vi "Shooter Button SUBVI.vi"   [LabVIEW 2013]
types:
  T1 = cluster{"Digital Input [1-16][0]":bool, "Digital Input [1-16][1]":bool, "Digital Input [1-16][2]":bool, "Digital Input [1-16][3]":bool, "Digital Input [1-16][4]":bool, "Digital Input [1-16][5]":bool, "Digital Input [1-16][6]":bool, "Digital Input [1-16][7]":bool, "Digital Input [1-16][8]":bool, "Digital Input [1-16][9]":bool, "Digital Input [1-16][10]":bool, "Digital Input [1-16][11]":bool, "Digital Input [1-16][12]":bool, "Digital Input [1-16][13]":bool, "Digital Input [1-16][14]":bool, "Digital Input [1-16][15]":bool}
  T2 = typedef "WPI_DigitalInputDevRef.ctl" = cluster{"DevStatus":errorcluster, "DIO Channel":T3, "Digital Module":T4}
  T3 = typedef "FPGA_DIOChannel.ctl" = enum8{"DIO 1", "DIO 2", "DIO 3", "DIO 4", "DIO 5", "DIO 6", "DIO 7", "DIO 8", "DIO 9", "DIO 10", "DIO 11", "DIO 12", "DIO 13", "DIO 14", "Invalid"}
  T4 = typedef "FPGA_TypedefDigitalModule.ctl" = enum16{"Digital Module 1", "Digital Module 2"}
  T5 = typedef "WPI_MotorControlDeviceRef.ctl" = cluster{"DeviceStatus":errorcluster, "Type":enum16{"PWM", "CAN"}, "PWM":cluster{"Digital Module":T4, "PWM Channel":T6, "DeadBand":T7}, "CAN":cluster{"Device Number":u8, "Control Mode":T8, "Semaphore":T9, "Max Vout":dbl}, "Invert":bool, "TransformRef":T10, "InvTransformRef":T10}
  T6 = typedef "FPGA_DIOPWMChannel.ctl" = enum8{"PWM 1", "PWM 2", "PWM 3", "PWM 4", "PWM 5", "PWM 6", "PWM 7", "PWM 8", "PWM 9", "PWM 10", "Invalid"}
  T7 = typedef "WPI_PWMDeadband.ctl" = cluster{"Name":string, "maxPositivePwm":i32, "minPositivePwm":i32, "centerPwm":i32, "maxNegativePwm":i32, "minNegativePwm":i32, "angularRange":u16}
  T8 = typedef "WPI_CANJaguar_ControlMode.ctl" = enum8{"Percent VBus", "Current", "Speed", "Position", "Voltage"}
  T9 = typedef "Semaphore RefNum" = refnum<k1>
  T10 = typedef "WPI_PWMTransform_ConPane.ctl" = refnum<vi>
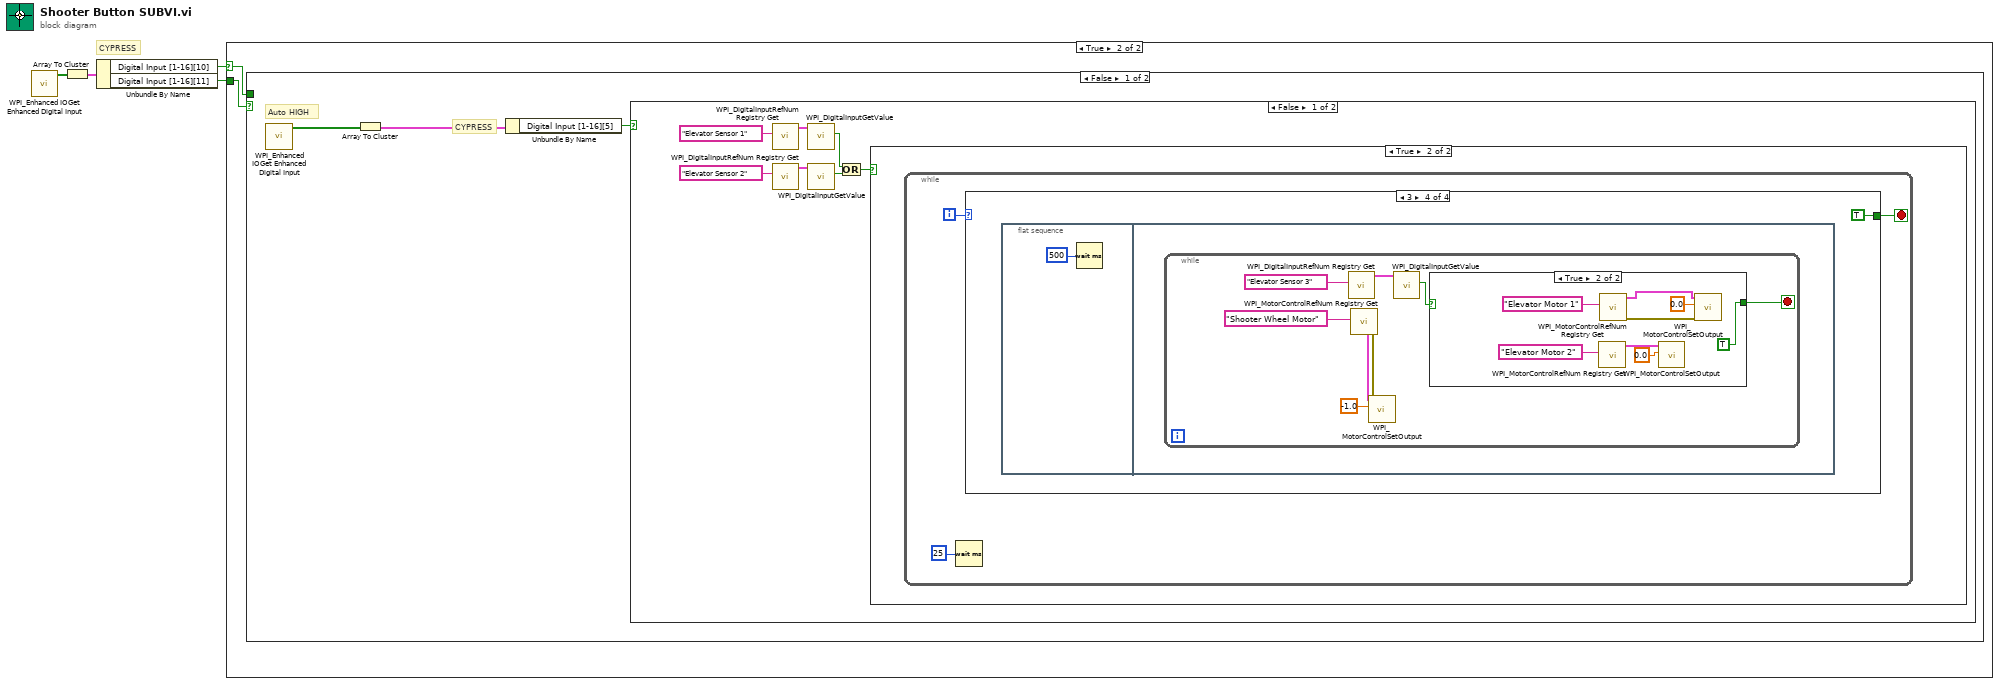
[diagram p0: block diagram]
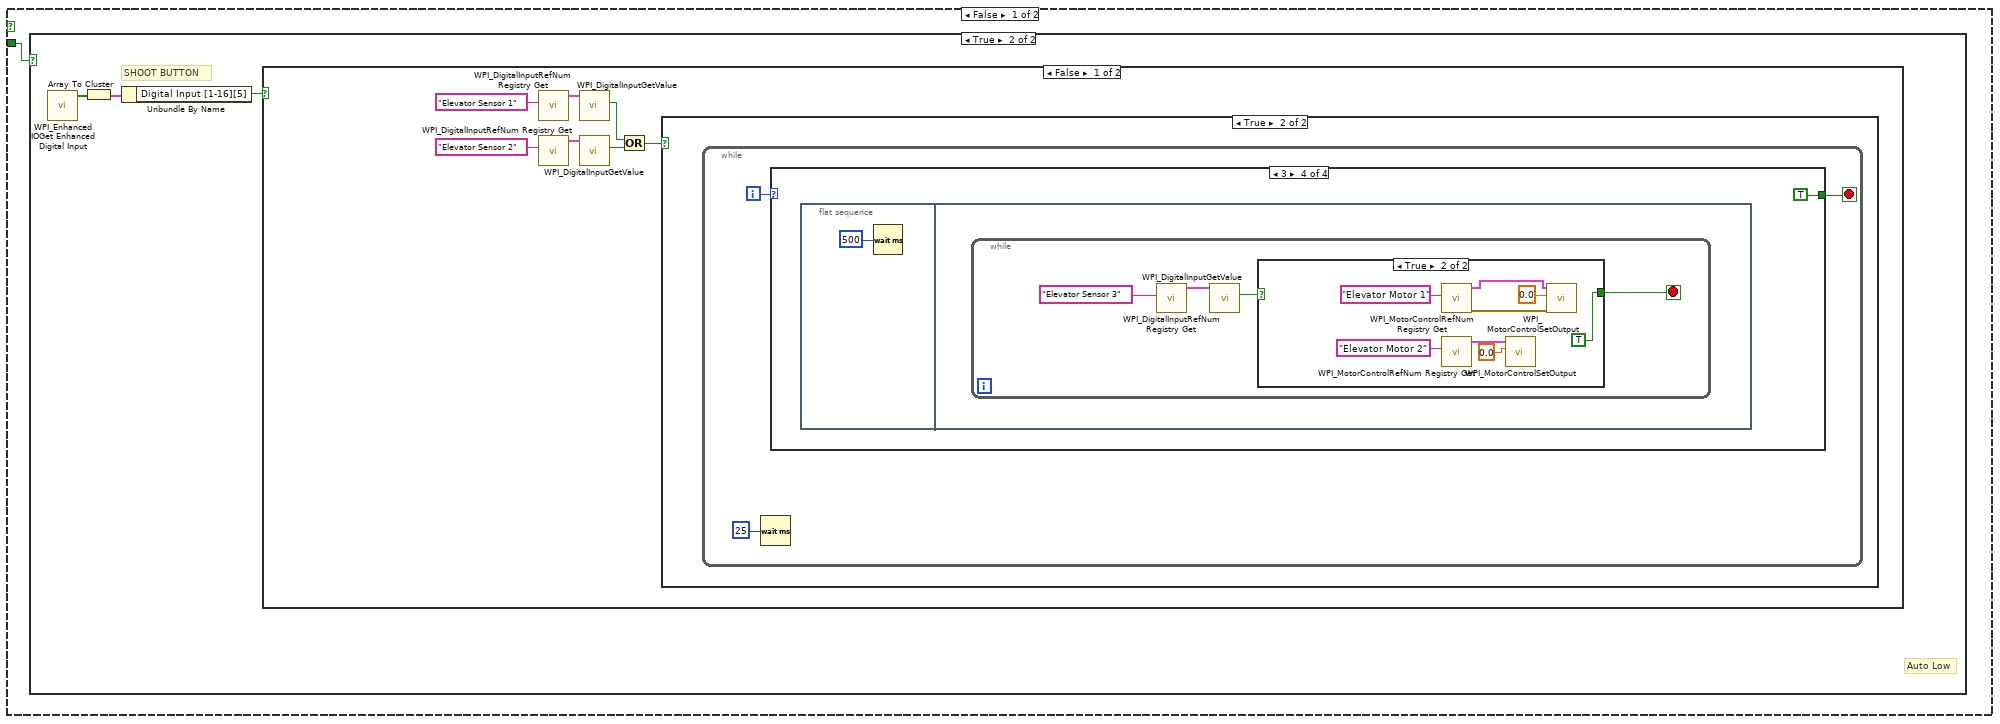
[diagram p2: hidden frame]
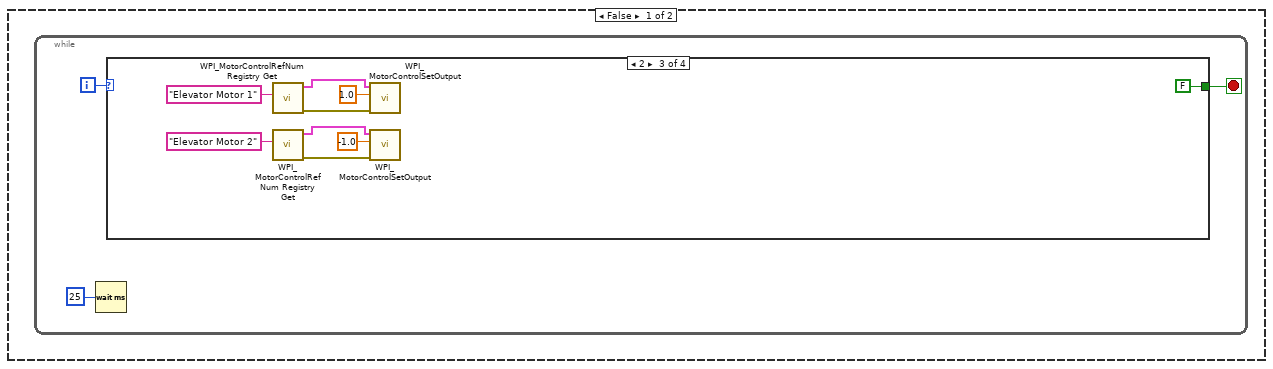
[diagram p4: hidden frame]
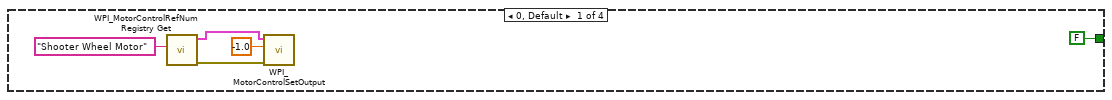
[diagram p5: hidden frame]
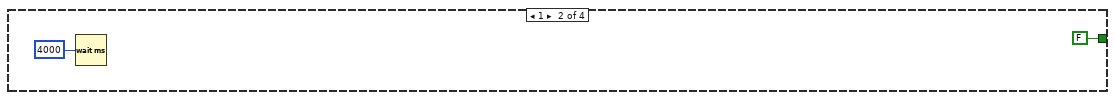
[diagram p6: hidden frame]
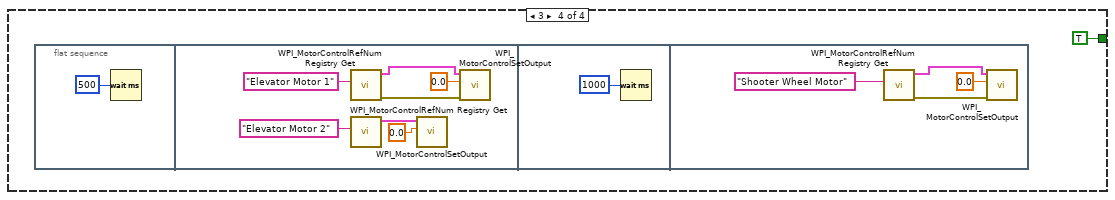
[diagram p7: hidden frame]
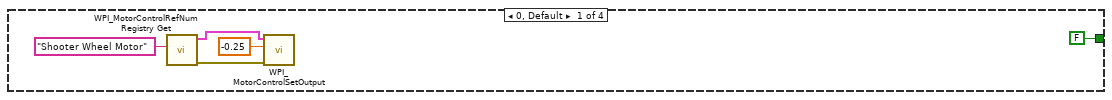
[diagram p8: hidden frame]
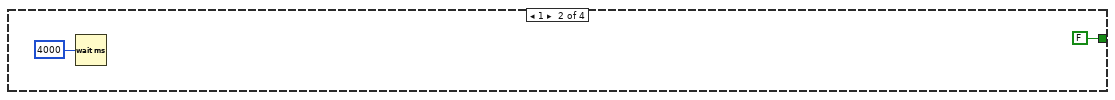
[diagram p9: hidden frame]
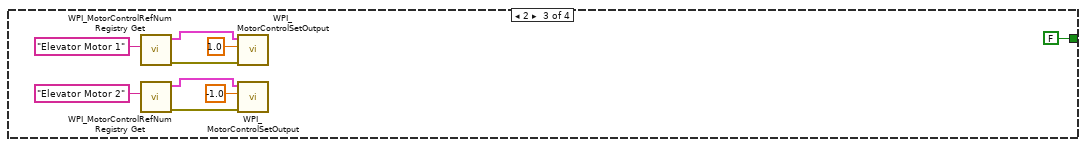
[diagram p10: hidden frame]
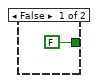
[diagram p11: hidden frame]
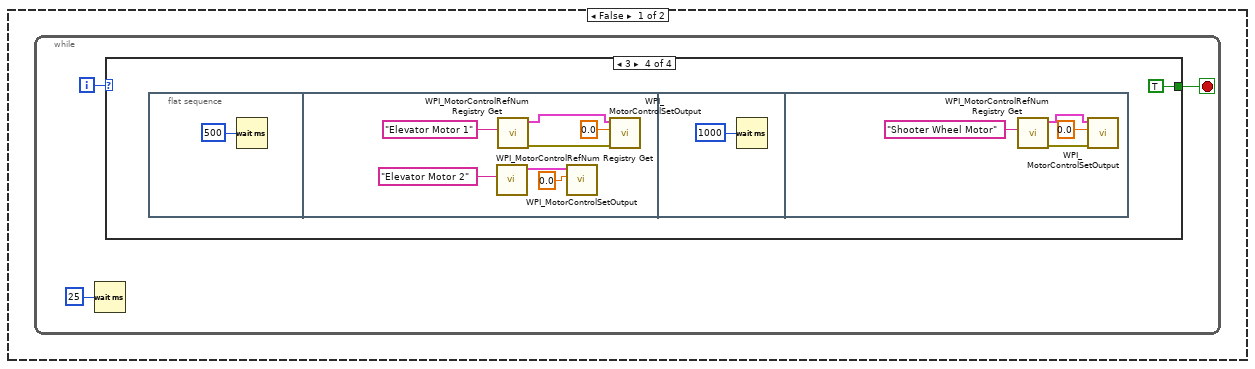
[diagram p13: hidden frame]
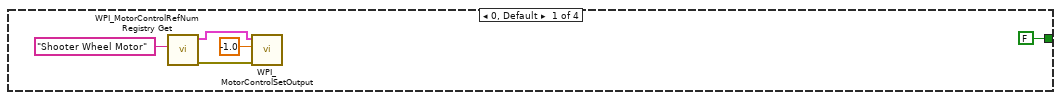
[diagram p14: hidden frame]
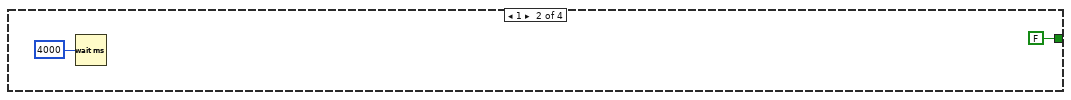
[diagram p15: hidden frame]
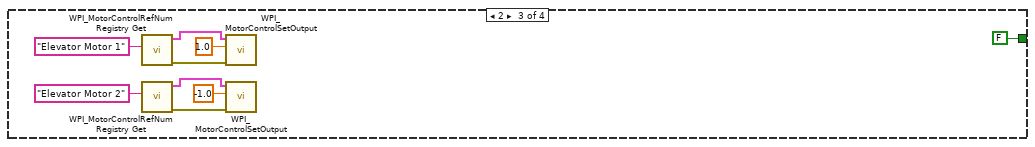
[diagram p16: hidden frame]
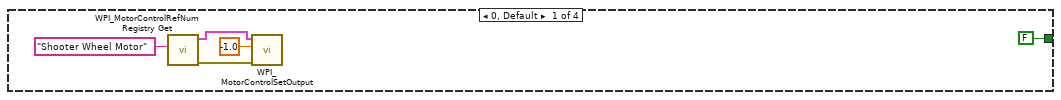
[diagram p17: hidden frame]
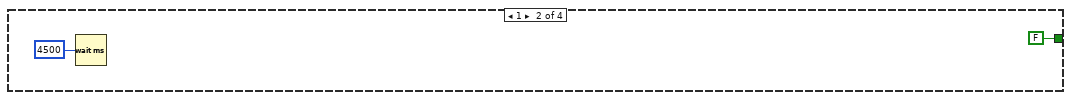
[diagram p18: hidden frame]
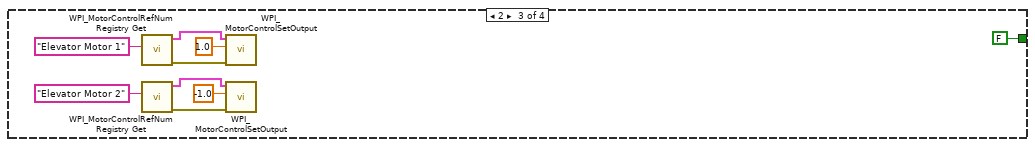
[diagram p19: hidden frame]
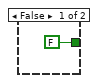
[diagram p20: hidden frame]
diagram:
  # "CYPRESS"
  n1 = call <vilib>:"WPI_Enhanced IOGet Enhanced Digital Input.vi"() -> ("Digital Input [1-16]"=w4:bool[])  [unwired: 10 in, 1 out]
  n2 = Array To Cluster(array=w4) -> (cluster=w3:T1)
  n3 = Unbundle By Name(w3) -> ("Digital Input [1-16][10]"=w2:bool, "Digital Input [1-16][11]"=w1:bool)
  n4 = case shown="True" w2 {
    selector: w2 -> [_ w83]
    tunnel: w1 -> [w5 w84]
    frame False {
      n5 = case shown="True" w5 {
        frame False {
        }
        frame True {
          # "Auto Low"
          # "SHOOT BUTTON"
          n6 = call <vilib>:"WPI_Enhanced IOGet Enhanced Digital Input.vi"() -> ("Digital Input [1-16]"=w8:bool[])  [unwired: 10 in, 1 out]
          n7 = Array To Cluster(array=w8) -> (cluster=w7:T1)
          n8 = Unbundle By Name(w7) -> ("Digital Input [1-16][5]"=w6:bool)
          n9 = case shown="False" w6 {
            frame False {
              n10 = call <vilib>:"WPI_DigitalInputRefNum Registry Get.vi"("refnum name"="Elevator Sensor 1") -> ("DigitalInputDevRef"=w14:T2)  [unwired: 9 in, 1 out]
              n11 = call <vilib>:"WPI_DigitalInputRefNum Registry Get.vi"("refnum name"="Elevator Sensor 2") -> ("DigitalInputDevRef"=w12:T2)  [unwired: 9 in, 1 out]
              n12 = call <vilib>:"WPI_DigitalInputGetValue.vi"("DigitalInputDevRef"=w14) -> ("Value"=w11:bool)  [unwired: 8 in, 2 out]
              n13 = call <vilib>:"WPI_DigitalInputGetValue.vi"("DigitalInputDevRef"=w12) -> ("Value"=w10:bool)  [unwired: 8 in, 2 out]
              n14 = Or(x=w11, y=w10) -> (x .or. y?=w9:bool)
              n15 = case shown="True" w9 {
                frame False {
                  n16 = while {
                    i -> [w18]
                    stop <- w16 stop-if-true
                    n17 = Wait (ms)(milliseconds to wait=u32 25) -> ()  [unwired: 1 out]
                    n18 = case shown="2" w18 {
                      tunnel: [FALSE FALSE FALSE TRUE] -> w16
                      frame 0, Default {
                        n19 = call <vilib>:"WPI_MotorControlRefNum Registry Get.vi"("refnum name"="Shooter Wheel Motor") -> ("error out"=w23:errorcluster, "MotorControlDevRef"=w22:T5)  [unwired: 9 in]
                        n20 = call <vilib>:"WPI_MotorControlSetOutput.vi"("error in (no error)"=w23, "Output"=-1.0, "MotorControlDevRef"=w22) -> ()  [unwired: 6 in, 3 out]
                      }
                      frame 1 {
                        n21 = Wait (ms)(milliseconds to wait=u32 4000) -> ()  [unwired: 1 out]
                      }
                      frame 2 {
                        n22 = call <vilib>:"WPI_MotorControlRefNum Registry Get.vi"("refnum name"="Elevator Motor 1") -> ("error out"=w30:errorcluster, "MotorControlDevRef"=w29:T5)  [unwired: 9 in]
                        n23 = call <vilib>:"WPI_MotorControlRefNum Registry Get.vi"("refnum name"="Elevator Motor 2") -> ("error out"=w34:errorcluster, "MotorControlDevRef"=w33:T5)  [unwired: 9 in]
                        n24 = call <vilib>:"WPI_MotorControlSetOutput.vi"("error in (no error)"=w30, "Output"=1.0, "MotorControlDevRef"=w29) -> ()  [unwired: 6 in, 3 out]
                        n25 = call <vilib>:"WPI_MotorControlSetOutput.vi"("error in (no error)"=w34, "Output"=-1.0, "MotorControlDevRef"=w33) -> ()  [unwired: 6 in, 3 out]
                      }
                      frame 3 {
                        n26 = flat-sequence {
                          frame #0 {
                            n27 = Wait (ms)(milliseconds to wait=u32 500) -> ()  [unwired: 1 out]
                          }
                          frame #1 {
                            n28 = call <vilib>:"WPI_MotorControlRefNum Registry Get.vi"("refnum name"="Elevator Motor 1") -> ("error out"=w42:errorcluster, "MotorControlDevRef"=w41:T5)  [unwired: 9 in]
                            n29 = call <vilib>:"WPI_MotorControlRefNum Registry Get.vi"("refnum name"="Elevator Motor 2") -> ("MotorControlDevRef"=w43:T5)  [unwired: 9 in, 1 out]
                            n30 = call <vilib>:"WPI_MotorControlSetOutput.vi"("Output"=0.0, "MotorControlDevRef"=w43) -> ()  [unwired: 7 in, 3 out]
                            n31 = call <vilib>:"WPI_MotorControlSetOutput.vi"("error in (no error)"=w42, "Output"=0.0, "MotorControlDevRef"=w41) -> ()  [unwired: 6 in, 3 out]
                          }
                          frame #2 {
                            n32 = Wait (ms)(milliseconds to wait=u32 1000) -> ()  [unwired: 1 out]
                          }
                          frame #3 {
                            n33 = call <vilib>:"WPI_MotorControlRefNum Registry Get.vi"("refnum name"="Shooter Wheel Motor") -> ("error out"=w48:errorcluster, "MotorControlDevRef"=w45:T5)  [unwired: 9 in]
                            n34 = call <vilib>:"WPI_MotorControlSetOutput.vi"("error in (no error)"=w48, "Output"=0.0, "MotorControlDevRef"=w45) -> ()  [unwired: 6 in, 3 out]
                          }
                        }
                      }
                    }
                  }
                }
                frame True {
                  n35 = while {
                    i -> [w51]
                    stop <- w49 stop-if-true
                    n36 = Wait (ms)(milliseconds to wait=u32 25) -> ()  [unwired: 1 out]
                    n37 = case shown="3" w51 {
                      tunnel: [FALSE FALSE FALSE TRUE] -> w49
                      frame 0, Default {
                        n38 = call <vilib>:"WPI_MotorControlRefNum Registry Get.vi"("refnum name"="Shooter Wheel Motor") -> ("error out"=w56:errorcluster, "MotorControlDevRef"=w55:T5)  [unwired: 9 in]
                        n39 = call <vilib>:"WPI_MotorControlSetOutput.vi"("error in (no error)"=w56, "Output"=-0.25, "MotorControlDevRef"=w55) -> ()  [unwired: 6 in, 3 out]
                      }
                      frame 1 {
                        n40 = Wait (ms)(milliseconds to wait=u32 4000) -> ()  [unwired: 1 out]
                      }
                      frame 2 {
                        n41 = call <vilib>:"WPI_MotorControlRefNum Registry Get.vi"("refnum name"="Elevator Motor 1") -> ("error out"=w63:errorcluster, "MotorControlDevRef"=w62:T5)  [unwired: 9 in]
                        n42 = call <vilib>:"WPI_MotorControlRefNum Registry Get.vi"("refnum name"="Elevator Motor 2") -> ("error out"=w67:errorcluster, "MotorControlDevRef"=w66:T5)  [unwired: 9 in]
                        n43 = call <vilib>:"WPI_MotorControlSetOutput.vi"("error in (no error)"=w63, "Output"=1.0, "MotorControlDevRef"=w62) -> ()  [unwired: 6 in, 3 out]
                        n44 = call <vilib>:"WPI_MotorControlSetOutput.vi"("error in (no error)"=w67, "Output"=-1.0, "MotorControlDevRef"=w66) -> ()  [unwired: 6 in, 3 out]
                      }
                      frame 3 {
                        n45 = flat-sequence {
                          frame #0 {
                            n46 = Wait (ms)(milliseconds to wait=u32 500) -> ()  [unwired: 1 out]
                          }
                          frame #1 {
                            n47 = while {
                              stop <- w70 stop-if-true
                              n48 = call <vilib>:"WPI_DigitalInputRefNum Registry Get.vi"("refnum name"="Elevator Sensor 3") -> ("DigitalInputDevRef"=w72:T2)  [unwired: 9 in, 1 out]
                              n49 = call <vilib>:"WPI_DigitalInputGetValue.vi"("DigitalInputDevRef"=w72) -> ("Value"=w71:bool)  [unwired: 8 in, 2 out]
                              n50 = case shown="True" w71 {
                                tunnel: [FALSE TRUE] -> w70
                                frame False {
                                }
                                frame True {
                                n51 = call <vilib>:"WPI_MotorControlRefNum Registry Get.vi"("refnum name"="Elevator Motor 1") -> ("error out"=w77:errorcluster, "MotorControlDevRef"=w78:T5)  [unwired: 9 in]
                                n52 = call <vilib>:"WPI_MotorControlRefNum Registry Get.vi"("refnum name"="Elevator Motor 2") -> ("MotorControlDevRef"=w76:T5)  [unwired: 9 in, 1 out]
                                n53 = call <vilib>:"WPI_MotorControlSetOutput.vi"("Output"=0.0, "MotorControlDevRef"=w76) -> ()  [unwired: 7 in, 3 out]
                                n54 = call <vilib>:"WPI_MotorControlSetOutput.vi"("error in (no error)"=w77, "Output"=0.0, "MotorControlDevRef"=w78) -> ()  [unwired: 6 in, 3 out]
                                }
                              }
                            }
                          }
                        }
                      }
                    }
                  }
                }
              }
            }
            frame True {
            }
          }
        }
      }
    }
    frame True {
      n55 = case shown="False" w84 {
        tunnel: w83 -> [_ _]
        frame False {
          # "CYPRESS"
          # "Auto HIGH"
          n56 = call <vilib>:"WPI_Enhanced IOGet Enhanced Digital Input.vi"() -> ("Digital Input [1-16]"=w87:bool[])  [unwired: 10 in, 1 out]
          n57 = Array To Cluster(array=w87) -> (cluster=w86:T1)
          n58 = Unbundle By Name(w86) -> ("Digital Input [1-16][5]"=w85:bool)
          n59 = case shown="False" w85 {
            frame False {
              n60 = call <vilib>:"WPI_DigitalInputRefNum Registry Get.vi"("refnum name"="Elevator Sensor 1") -> ("DigitalInputDevRef"=w93:T2)  [unwired: 9 in, 1 out]
              n61 = call <vilib>:"WPI_DigitalInputRefNum Registry Get.vi"("refnum name"="Elevator Sensor 2") -> ("DigitalInputDevRef"=w91:T2)  [unwired: 9 in, 1 out]
              n62 = call <vilib>:"WPI_DigitalInputGetValue.vi"("DigitalInputDevRef"=w93) -> ("Value"=w90:bool)  [unwired: 8 in, 2 out]
              n63 = call <vilib>:"WPI_DigitalInputGetValue.vi"("DigitalInputDevRef"=w91) -> ("Value"=w89:bool)  [unwired: 8 in, 2 out]
              n64 = Or(x=w90, y=w89) -> (x .or. y?=w88:bool)
              n65 = case shown="True" w88 {
                frame False {
                  n66 = while {
                    i -> [w97]
                    stop <- w95 stop-if-true
                    n67 = Wait (ms)(milliseconds to wait=u32 25) -> ()  [unwired: 1 out]
                    n68 = case shown="3" w97 {
                      tunnel: [FALSE FALSE FALSE TRUE] -> w95
                      frame 0, Default {
                        n69 = call <vilib>:"WPI_MotorControlRefNum Registry Get.vi"("refnum name"="Shooter Wheel Motor") -> ("error out"=w102:errorcluster, "MotorControlDevRef"=w101:T5)  [unwired: 9 in]
                        n70 = call <vilib>:"WPI_MotorControlSetOutput.vi"("error in (no error)"=w102, "Output"=-1.0, "MotorControlDevRef"=w101) -> ()  [unwired: 6 in, 3 out]
                      }
                      frame 1 {
                        n71 = Wait (ms)(milliseconds to wait=u32 4000) -> ()  [unwired: 1 out]
                      }
                      frame 2 {
                        n72 = call <vilib>:"WPI_MotorControlRefNum Registry Get.vi"("refnum name"="Elevator Motor 1") -> ("error out"=w109:errorcluster, "MotorControlDevRef"=w108:T5)  [unwired: 9 in]
                        n73 = call <vilib>:"WPI_MotorControlRefNum Registry Get.vi"("refnum name"="Elevator Motor 2") -> ("error out"=w113:errorcluster, "MotorControlDevRef"=w112:T5)  [unwired: 9 in]
                        n74 = call <vilib>:"WPI_MotorControlSetOutput.vi"("error in (no error)"=w109, "Output"=1.0, "MotorControlDevRef"=w108) -> ()  [unwired: 6 in, 3 out]
                        n75 = call <vilib>:"WPI_MotorControlSetOutput.vi"("error in (no error)"=w113, "Output"=-1.0, "MotorControlDevRef"=w112) -> ()  [unwired: 6 in, 3 out]
                      }
                      frame 3 {
                        n76 = flat-sequence {
                          frame #0 {
                            n77 = Wait (ms)(milliseconds to wait=u32 500) -> ()  [unwired: 1 out]
                          }
                          frame #1 {
                            n78 = call <vilib>:"WPI_MotorControlRefNum Registry Get.vi"("refnum name"="Elevator Motor 2") -> ("MotorControlDevRef"=w122:T5)  [unwired: 9 in, 1 out]
                            n79 = call <vilib>:"WPI_MotorControlRefNum Registry Get.vi"("refnum name"="Elevator Motor 1") -> ("error out"=w121:errorcluster, "MotorControlDevRef"=w120:T5)  [unwired: 9 in]
                            n80 = call <vilib>:"WPI_MotorControlSetOutput.vi"("Output"=0.0, "MotorControlDevRef"=w122) -> ()  [unwired: 7 in, 3 out]
                            n81 = call <vilib>:"WPI_MotorControlSetOutput.vi"("error in (no error)"=w121, "Output"=0.0, "MotorControlDevRef"=w120) -> ()  [unwired: 6 in, 3 out]
                          }
                          frame #2 {
                            n82 = Wait (ms)(milliseconds to wait=u32 1000) -> ()  [unwired: 1 out]
                          }
                          frame #3 {
                            n83 = call <vilib>:"WPI_MotorControlRefNum Registry Get.vi"("refnum name"="Shooter Wheel Motor") -> ("error out"=w127:errorcluster, "MotorControlDevRef"=w124:T5)  [unwired: 9 in]
                            n84 = call <vilib>:"WPI_MotorControlSetOutput.vi"("error in (no error)"=w127, "Output"=0.0, "MotorControlDevRef"=w124) -> ()  [unwired: 6 in, 3 out]
                          }
                        }
                      }
                    }
                  }
                }
                frame True {
                  n85 = while {
                    i -> [w130]
                    stop <- w128 stop-if-true
                    n86 = Wait (ms)(milliseconds to wait=u32 25) -> ()  [unwired: 1 out]
                    n87 = case shown="3" w130 {
                      tunnel: [FALSE FALSE FALSE TRUE] -> w128
                      frame 0, Default {
                        n88 = call <vilib>:"WPI_MotorControlRefNum Registry Get.vi"("refnum name"="Shooter Wheel Motor") -> ("error out"=w135:errorcluster, "MotorControlDevRef"=w134:T5)  [unwired: 9 in]
                        n89 = call <vilib>:"WPI_MotorControlSetOutput.vi"("error in (no error)"=w135, "Output"=-1.0, "MotorControlDevRef"=w134) -> ()  [unwired: 6 in, 3 out]
                      }
                      frame 1 {
                        n90 = Wait (ms)(milliseconds to wait=u32 4500) -> ()  [unwired: 1 out]
                      }
                      frame 2 {
                        n91 = call <vilib>:"WPI_MotorControlRefNum Registry Get.vi"("refnum name"="Elevator Motor 1") -> ("error out"=w142:errorcluster, "MotorControlDevRef"=w141:T5)  [unwired: 9 in]
                        n92 = call <vilib>:"WPI_MotorControlRefNum Registry Get.vi"("refnum name"="Elevator Motor 2") -> ("error out"=w146:errorcluster, "MotorControlDevRef"=w145:T5)  [unwired: 9 in]
                        n93 = call <vilib>:"WPI_MotorControlSetOutput.vi"("error in (no error)"=w142, "Output"=1.0, "MotorControlDevRef"=w141) -> ()  [unwired: 6 in, 3 out]
                        n94 = call <vilib>:"WPI_MotorControlSetOutput.vi"("error in (no error)"=w146, "Output"=-1.0, "MotorControlDevRef"=w145) -> ()  [unwired: 6 in, 3 out]
                      }
                      frame 3 {
                        n95 = flat-sequence {
                          frame #0 {
                            n96 = Wait (ms)(milliseconds to wait=u32 500) -> ()  [unwired: 1 out]
                          }
                          frame #1 {
                            n97 = while {
                              stop <- w153 stop-if-true
                              n98 = call <vilib>:"WPI_DigitalInputRefNum Registry Get.vi"("refnum name"="Elevator Sensor 3") -> ("DigitalInputDevRef"=w155:T2)  [unwired: 9 in, 1 out]
                              n99 = call <vilib>:"WPI_MotorControlRefNum Registry Get.vi"("refnum name"="Shooter Wheel Motor") -> ("error out"=w149:errorcluster, "MotorControlDevRef"=w150:T5)  [unwired: 9 in]
                              n100 = call <vilib>:"WPI_MotorControlSetOutput.vi"("error in (no error)"=w149, "Output"=-1.0, "MotorControlDevRef"=w150) -> ()  [unwired: 6 in, 3 out]
                              n101 = call <vilib>:"WPI_DigitalInputGetValue.vi"("DigitalInputDevRef"=w155) -> ("Value"=w154:bool)  [unwired: 8 in, 2 out]
                              n102 = case shown="True" w154 {
                                tunnel: [FALSE TRUE] -> w153
                                frame False {
                                }
                                frame True {
                                n103 = call <vilib>:"WPI_MotorControlRefNum Registry Get.vi"("refnum name"="Elevator Motor 2") -> ("MotorControlDevRef"=w159:T5)  [unwired: 9 in, 1 out]
                                n104 = call <vilib>:"WPI_MotorControlRefNum Registry Get.vi"("refnum name"="Elevator Motor 1") -> ("error out"=w160:errorcluster, "MotorControlDevRef"=w161:T5)  [unwired: 9 in]
                                n105 = call <vilib>:"WPI_MotorControlSetOutput.vi"("Output"=0.0, "MotorControlDevRef"=w159) -> ()  [unwired: 7 in, 3 out]
                                n106 = call <vilib>:"WPI_MotorControlSetOutput.vi"("error in (no error)"=w160, "Output"=0.0, "MotorControlDevRef"=w161) -> ()  [unwired: 6 in, 3 out]
                                }
                              }
                            }
                          }
                        }
                      }
                    }
                  }
                }
              }
            }
            frame True {
            }
          }
        }
        frame True {
          # "AUTO MEDIUM"
          n107 = call <vilib>:"WPI_Enhanced IOGet Enhanced Digital Input.vi"() -> ("Digital Input [1-16]"=w167:bool[])  [unwired: 10 in, 1 out]
          n108 = Array To Cluster(array=w167) -> (cluster=w168:T1)
          n109 = Unbundle By Name(w168) -> ("Digital Input [1-16][5]"=w166:bool)
          n110 = case shown="False" w166 {
            frame False {
              n111 = call <vilib>:"WPI_DigitalInputRefNum Registry Get.vi"("refnum name"="Elevator Sensor 1") -> ("DigitalInputDevRef"=w174:T2)  [unwired: 9 in, 1 out]
              n112 = call <vilib>:"WPI_DigitalInputRefNum Registry Get.vi"("refnum name"="Elevator Sensor 2") -> ("DigitalInputDevRef"=w172:T2)  [unwired: 9 in, 1 out]
              n113 = call <vilib>:"WPI_DigitalInputGetValue.vi"("DigitalInputDevRef"=w174) -> ("Value"=w171:bool)  [unwired: 8 in, 2 out]
              n114 = call <vilib>:"WPI_DigitalInputGetValue.vi"("DigitalInputDevRef"=w172) -> ("Value"=w170:bool)  [unwired: 8 in, 2 out]
              n115 = Or(x=w171, y=w170) -> (x .or. y?=w169:bool)
              n116 = case shown="False" w169 {
                frame False {
                  n117 = while {
                    i -> [w178]
                    stop <- w176 stop-if-true
                    n118 = Wait (ms)(milliseconds to wait=u32 25) -> ()  [unwired: 1 out]
                    n119 = case shown="0, Default" w178 {
                      tunnel: [FALSE FALSE FALSE TRUE] -> w176
                      frame 0, Default {
                        n120 = call <vilib>:"WPI_MotorControlRefNum Registry Get.vi"("refnum name"="Shooter Wheel Motor") -> ("error out"=w183:errorcluster, "MotorControlDevRef"=w182:T5)  [unwired: 9 in]
                        n121 = call <vilib>:"WPI_MotorControlSetOutput.vi"("error in (no error)"=w183, "Output"=-0.5, "MotorControlDevRef"=w182) -> ()  [unwired: 6 in, 3 out]
                      }
                      frame 1 {
                        n122 = Wait (ms)(milliseconds to wait=u32 4000) -> ()  [unwired: 1 out]
                      }
                      frame 2 {
                        n123 = call <vilib>:"WPI_MotorControlRefNum Registry Get.vi"("refnum name"="Elevator Motor 1") -> ("error out"=w190:errorcluster, "MotorControlDevRef"=w189:T5)  [unwired: 9 in]
                        n124 = call <vilib>:"WPI_MotorControlRefNum Registry Get.vi"("refnum name"="Elevator Motor 2") -> ("error out"=w194:errorcluster, "MotorControlDevRef"=w193:T5)  [unwired: 9 in]
                        n125 = call <vilib>:"WPI_MotorControlSetOutput.vi"("error in (no error)"=w190, "Output"=1.0, "MotorControlDevRef"=w189) -> ()  [unwired: 6 in, 3 out]
                        n126 = call <vilib>:"WPI_MotorControlSetOutput.vi"("error in (no error)"=w194, "Output"=-1.0, "MotorControlDevRef"=w193) -> ()  [unwired: 6 in, 3 out]
                      }
                      frame 3 {
                        n127 = flat-sequence {
                          frame #0 {
                            n128 = Wait (ms)(milliseconds to wait=u32 500) -> ()  [unwired: 1 out]
                          }
                          frame #1 {
                            n129 = call <vilib>:"WPI_MotorControlRefNum Registry Get.vi"("refnum name"="Elevator Motor 1") -> ("error out"=w203:errorcluster, "MotorControlDevRef"=w202:T5)  [unwired: 9 in]
                            n130 = call <vilib>:"WPI_MotorControlRefNum Registry Get.vi"("refnum name"="Elevator Motor 2") -> ("error out"=w197:errorcluster, "MotorControlDevRef"=w204:T5)  [unwired: 9 in]
                            n131 = call <vilib>:"WPI_MotorControlSetOutput.vi"("error in (no error)"=w203, "Output"=0.0, "MotorControlDevRef"=w202) -> ()  [unwired: 6 in, 3 out]
                            n132 = call <vilib>:"WPI_MotorControlSetOutput.vi"("error in (no error)"=w197, "Output"=0.0, "MotorControlDevRef"=w204) -> ()  [unwired: 6 in, 3 out]
                          }
                          frame #2 {
                            n133 = Wait (ms)(milliseconds to wait=u32 1000) -> ()  [unwired: 1 out]
                          }
                          frame #3 {
                            n134 = call <vilib>:"WPI_MotorControlRefNum Registry Get.vi"("refnum name"="Shooter Wheel Motor") -> ("error out"=w209:errorcluster, "MotorControlDevRef"=w206:T5)  [unwired: 9 in]
                            n135 = call <vilib>:"WPI_MotorControlSetOutput.vi"("error in (no error)"=w209, "Output"=0.0, "MotorControlDevRef"=w206) -> ()  [unwired: 6 in, 3 out]
                          }
                        }
                      }
                    }
                  }
                }
                frame True {
                  n136 = while {
                    i -> [w212]
                    stop <- w210 stop-if-true
                    n137 = Wait (ms)(milliseconds to wait=u32 25) -> ()  [unwired: 1 out]
                    n138 = case shown="3" w212 {
                      tunnel: [FALSE FALSE FALSE TRUE] -> w210
                      frame 0, Default {
                        n139 = call <vilib>:"WPI_MotorControlRefNum Registry Get.vi"("refnum name"="Shooter Wheel Motor") -> ("error out"=w217:errorcluster, "MotorControlDevRef"=w216:T5)  [unwired: 9 in]
                        n140 = call <vilib>:"WPI_MotorControlSetOutput.vi"("error in (no error)"=w217, "Output"=-1.0, "MotorControlDevRef"=w216) -> ()  [unwired: 6 in, 3 out]
                      }
                      frame 1 {
                        n141 = Wait (ms)(milliseconds to wait=u32 4000) -> ()  [unwired: 1 out]
                      }
                      frame 2 {
                        n142 = call <vilib>:"WPI_MotorControlRefNum Registry Get.vi"("refnum name"="Elevator Motor 1") -> ("error out"=w224:errorcluster, "MotorControlDevRef"=w223:T5)  [unwired: 9 in]
                        n143 = call <vilib>:"WPI_MotorControlRefNum Registry Get.vi"("refnum name"="Elevator Motor 2") -> ("error out"=w228:errorcluster, "MotorControlDevRef"=w227:T5)  [unwired: 9 in]
                        n144 = call <vilib>:"WPI_MotorControlSetOutput.vi"("error in (no error)"=w224, "Output"=1.0, "MotorControlDevRef"=w223) -> ()  [unwired: 6 in, 3 out]
                        n145 = call <vilib>:"WPI_MotorControlSetOutput.vi"("error in (no error)"=w228, "Output"=-1.0, "MotorControlDevRef"=w227) -> ()  [unwired: 6 in, 3 out]
                      }
                      frame 3 {
                        n146 = flat-sequence {
                          frame #0 {
                            n147 = Wait (ms)(milliseconds to wait=u32 500) -> ()  [unwired: 1 out]
                          }
                          frame #1 {
                            n148 = while {
                              stop <- w232 stop-if-true
                              n149 = call <vilib>:"WPI_DigitalInputRefNum Registry Get.vi"("refnum name"="Elevator Sensor 3") -> ("error out"=w231:errorcluster, "DigitalInputDevRef"=w234:T2)  [unwired: 9 in]
                              n150 = call <vilib>:"WPI_DigitalInputGetValue.vi"("error in (no error)"=w231, "DigitalInputDevRef"=w234) -> ("Value"=w233:bool)  [unwired: 7 in, 2 out]
                              n151 = case shown="True" w233 {
                                tunnel: [FALSE TRUE] -> w232
                                frame False {
                                }
                                frame True {
                                n152 = call <vilib>:"WPI_MotorControlRefNum Registry Get.vi"("refnum name"="Elevator Motor 1") -> ("error out"=w239:errorcluster, "MotorControlDevRef"=w240:T5)  [unwired: 9 in]
                                n153 = call <vilib>:"WPI_MotorControlRefNum Registry Get.vi"("refnum name"="Elevator Motor 2") -> ("MotorControlDevRef"=w238:T5)  [unwired: 9 in, 1 out]
                                n154 = call <vilib>:"WPI_MotorControlSetOutput.vi"("Output"=0.0, "MotorControlDevRef"=w238) -> ()  [unwired: 7 in, 3 out]
                                n155 = call <vilib>:"WPI_MotorControlSetOutput.vi"("error in (no error)"=w239, "Output"=0.0, "MotorControlDevRef"=w240) -> ()  [unwired: 6 in, 3 out]
                                }
                              }
                            }
                          }
                        }
                      }
                    }
                  }
                }
              }
            }
            frame True {
            }
          }
        }
      }
    }
  }
